vi "ConvolveFile.vi"(11 "Old Files":T1[](array[typedef])) -> ()   [LabVIEW 2025]
uses:
  Curtin1_Label.ctl
panel:
  in  "Save":bool=TRUE
  out "ratio":dbl format="%0.2e"
  in  "Musical Piece":enum32{"Default", "Advanced"}(tab)
  in  "Path":path
  in  "Play 3":bool
  in  "Sampling rate":u16=48000
  out "FRF":cluster{"t0":dbl, "dt":dbl, dbl[]}[](graph)=[{"t0"=0.0, "dt"=0.732421875, array[13995 elements]}, {"t0"=0.0, "dt"=0.732421875, array[13995 elements]}]
  out "PointIdx":i32=359
  out "CursLoc":cluster{"X":dbl, "Y":dbl}={"X"=262.939453125, "Y"=26.045098132964196}
  out "CursIdx":i32=1
  in  "Play 2":bool
  in  "Play":bool
  in  "Save Convolve":bool
  in  "Instruments":u16(ring) items=["1727 Kreutzer Vengerov Strad 01 H.AvC"]
  # "Left ear is original\nRight ear is modified"
  # "Tchaikovsky Violin Concerto run"
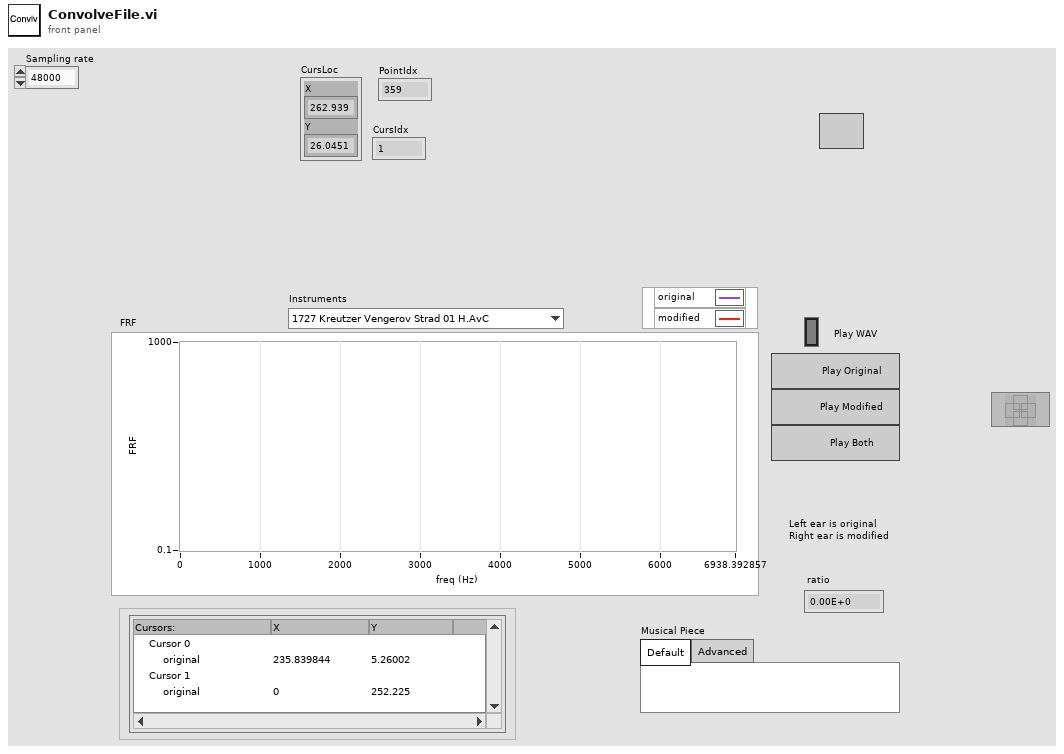
[diagram p1: front panel]
types:
  T1 = typedef "Curtin1_Label.ctl" = cluster{"Show?":bool, "Name":string, "Color":u32, "Path":path, "Show Notes":bool}
  T2 = typedef "PreferencesControl.ctl" = cluster{"Name of test":string, "Date":timestamp, "Location":string, "Template":string, "Soundcard":string, "resolution":u16, "Sampling rate":u16, "Ch1 Gain ":dbl, "Ch2 Gain":dbl, "Sample time (s)":dbl, "Pre-trigger (s)":dbl, "Hammer Threshold":dbl, "Positions":i16, "Taps/Position":i16, "Set Names":string, "Freq resolution":dbl, "Hammer cutoff":dbl, "Mic cutoff":dbl, "Double bounce ":dbl, "Hammer Cal":dbl, "dB Offset":dbl, "Accel Cal":dbl, "Vibrometer Cal":dbl, "Mic Cal":dbl, "Output":u16, "Voltage Cal":dbl, "Vibrometer Port":refnum<visa-resource-name>, "Range":u16, "High Pass":u16, "Bandwidth":u16, "X Range":cluster{"Minimum":dbl, "Maximum":dbl, "Increment":dbl, "Minor Increment":dbl, "Start":dbl}[], "Y Range":cluster{"Minimum":dbl, "Maximum":dbl, "Increment":dbl, "Minor Increment":dbl, "Start":dbl}[], "dB Spread":dbl, "Trigger":u16, "Ch_1":u8, "Ch_2":u8, "flip?":bool, "60Hz":bool, "Time offset":dbl, "Piezo Cal":dbl, "Default Notes":string, "Tom":bool}
  T3 = typedef "LVCursorListTypeDef.ctl" = cluster{"Name":string, "Color":u32, "Style":u8, "Point Style":u8, "Name Visible":bool, "Allow Drag":bool, "Cursor Mode":u32, "Plot":i32, "Index":i32, "Position":cluster{"X":dbl, "Y":dbl}, "X Scale":u32, "Y Scale":u32, "Watch Plots":i32[], "Watch All Plots":bool, "Plot Area":i32, "Label Offset":cluster{"X":dbl, "Y":dbl}}[]
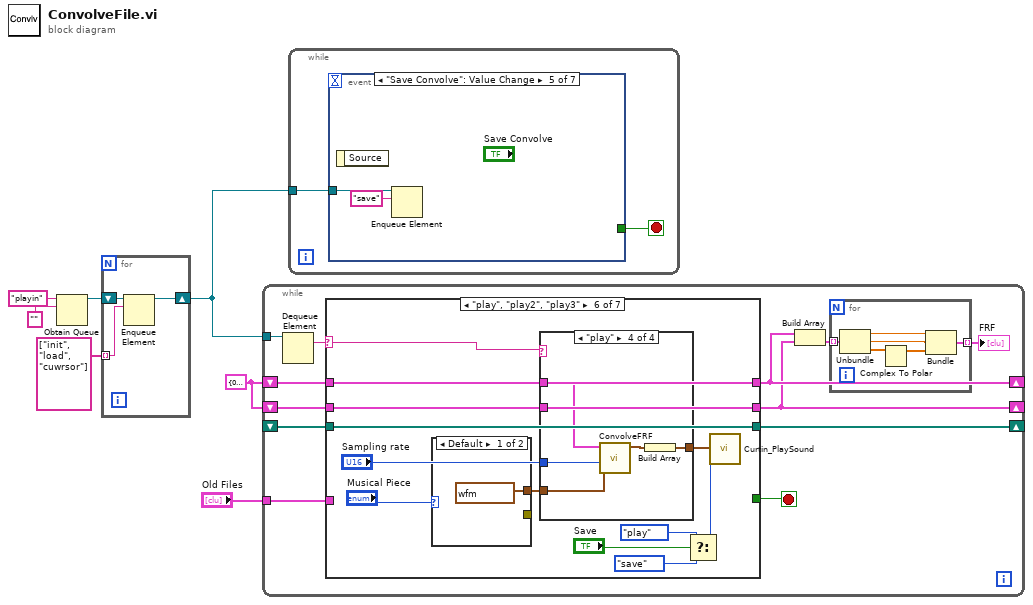
[diagram p0: block diagram]
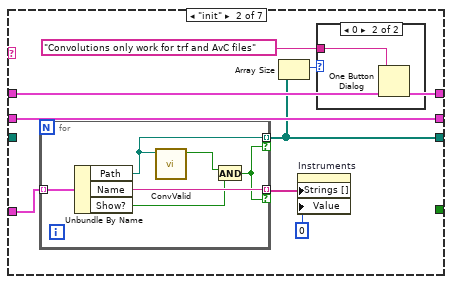
[diagram p3: hidden frame]
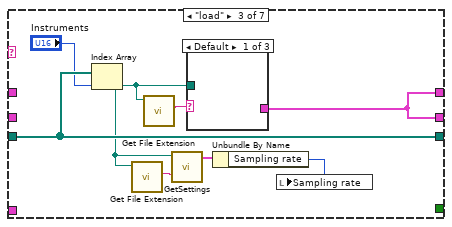
[diagram p5: hidden frame]
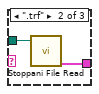
[diagram p6: hidden frame]
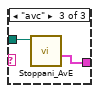
[diagram p7: hidden frame]
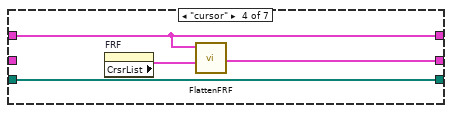
[diagram p8: hidden frame]
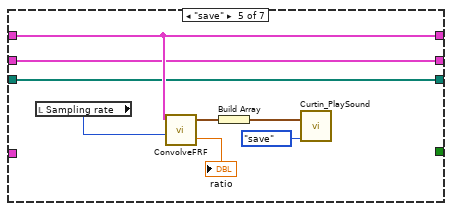
[diagram p9: hidden frame]
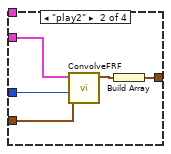
[diagram p11: hidden frame]
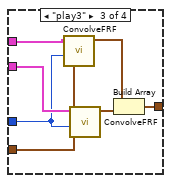
[diagram p12: hidden frame]
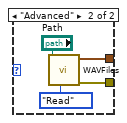
[diagram p13: hidden frame]
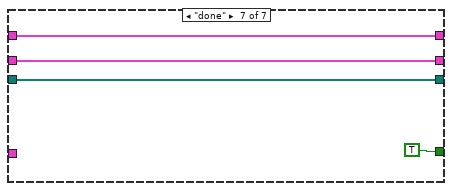
[diagram p14: hidden frame]
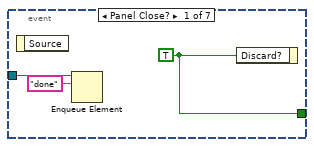
[diagram p15: hidden frame]
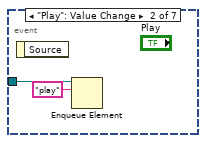
[diagram p16: hidden frame]
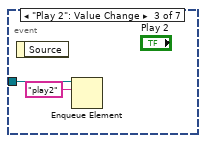
[diagram p17: hidden frame]
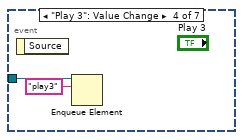
[diagram p18: hidden frame]
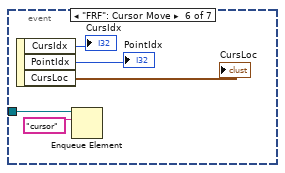
[diagram p19: hidden frame]
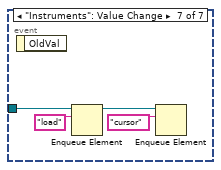
[diagram p20: hidden frame]
diagram:
  w1 = cluster{"t0":dbl, "dt":dbl, "Y":cdb[]} {"t0"=0.0, "dt"=0.0, "Y"=[]} ("Complex FRF")
  n1 = Obtain Queue(name (unnamed)="playin", element data type="" ("element")) -> (queue out=w7:refnum<queue>)  [unwired: 3 in, 2 out]
  n2 = for {
    shift-right: [w9] -> w6
    shift-left: w7 -> [w10]
    tunnel: string[] ["init", "load", "cuwrsor"] -> [w8] mode=indexing
    n3 = Enqueue Element(queue=w10, element=w8) -> (queue out=w9:refnum<queue>)  [unwired: 2 in, 2 out]
  }
  n4 = while {
    tunnel: w6 -> [w22]
    shift-right: [w16] -> _
    shift-left: w1 -> [w19]
    shift-right: [w15] -> _
    shift-left: w1 -> [w18]
    tunnel: "Old Files" -> [w13]
    shift-right: [w12] -> _
    shift-left: _ -> [w11]
    stop <- w20 stop-if-true
    n5 = Dequeue Element(queue=w22) -> (element=w21:string)  [unwired: 2 in, 3 out]
    n6 = case shown="\"play\", \"play2\", \"play3\"" w21 {
      selector: w21 -> [_ _ _ _ _ w76 _]
      tunnel: [_ _ _ _ _ _ TRUE] -> w20
      tunnel: [w31 w39 w54 w61 w69 w75 w107] -> w16
      tunnel: w19 -> [w31 w39 _ w61 w69 w75 w107]
      tunnel: w18 -> [w30 w38 _ _ w67 w80 w106]
      tunnel: [w30 w38 w54 w59 w67 w80 w106] -> w15
      tunnel: w13 -> [_ w35 _ _ _ _ _]
      tunnel: [w29 w34 w53 w62 w66 w79 w105] -> w12
      tunnel: w11 -> [w29 _ w53 w62 w66 w79 w105]
      frame Default {
      }
      frame "init" {
        n7 = for {
          tunnel: [w46] -> w37 mode=indexing if=w42
          tunnel: [w44] -> w34 mode=indexing if=w42
          tunnel: w35 -> [w45] mode=indexing
          n8 = Unbundle By Name(w45) -> ("Path"=w44:path, "Name"=w46:string, "Show?"=w43:bool)
          n9 = call "ConvValid.vi"("Path"=w44) -> ("Valid"=w41:bool)  [unwired: 10 in]
          n10 = And(x=w41, y=w43) -> (x .and. y?=w42:bool)
        }
        n11 = Array Size(array=w34) -> (size(s)=w33:i32)
        n12 = property on="Instruments" class="Ring (strict)"("Strings []"=w37, "Value"=0) -> ()  [unwired: 2 in, 2 out]
        n13 = case shown="0" w33 {
          tunnel: "Convolutions only work for trf and AvC files" ("element") -> [_ w40]
          frame Default {
          }
          frame 0 {
            n14 = One Button Dialog(message=w40) -> ()  [unwired: 1 in, 1 out]
          }
        }
      }
      frame "load" {
        n15 = Index Array(array=w53, index="Instruments") -> (element=w48:path)
        n16 = call <vilib>:"Get File Extension.vi"("file"=w48) -> ("lowercase file extension"=w52:string)  [unwired: 6 in, 4 out]
        n17 = call <vilib>:"Get File Extension.vi"("file"=w48) -> ("lowercase file extension"=w47:string)  [unwired: 6 in, 4 out]
        n18 = call "GetSettings.vi"("lowercase file extension"=w52, "wavform file"=w48) -> ("Settings"=w51:T2)  [unwired: 8 in, 1 out]
        n19 = case shown="Default" w47 {
          tunnel: [_ w56 w57] -> w54
          tunnel: w48 -> [_ w55 w58]
          frame Default {
          }
          frame ".trf" {
            n20 = call "Stoppani File Read.vi"("String in"=w55) -> ("Complex FRF"=w56:cluster{"t0":dbl, "dt":dbl, "Y":cdb[]})  [unwired: 2 in, 3 out]
          }
          frame "avc" {
            n21 = call "Stoppani_AvE.vi"("file (use dialog)"=w58) -> ("Complex FRF"=w57:cluster{"t0":dbl, "df":dbl, "Y":cdb[]})  [unwired: 7 in, 3 out]
          }
        }
        n22 = Unbundle By Name(w51) -> ("Sampling rate"=w50:u16)
        n23 = local write "Sampling rate"(w50) -> ()
      }
      frame "cursor" {
        n24 = property on="FRF" class="WFGraph (strict)"() -> ("CrsrList"=w60:T3)  [unwired: 2 in, 2 out]
        n25 = call "FlattenFRF.vi"("CrsrList"=w60, "Complex FRF in"=w61) -> ("Complex FRF out"=w59:cluster{"t0":dbl, "dt":dbl, "Y":cdb[]})  [unwired: 9 in]
      }
      frame "save" {
        n26 = local read "Sampling rate"() -> (w65:u16)
        n27 = call "ConvolveFRF.vi"("Sampling rate"=w65, "Complex FRF"=w69) -> ("Convolution"=w68:waveform(dbl), "ratio"=→"ratio":dbl)  [unwired: 6 in, 2 out]
        n28 = Build Array(w68) -> (w70:waveform(dbl)[])
        n29 = call "Curtin_PlaySound.vi"("Task"=enum16{"play", "save"}."save", "all waveforms"=w70) -> ()  [unwired: 9 in, 1 out]
      }
      frame "play", "play2", "play3" {
        n30 = case shown="Default" "Musical Piece" {
          tunnel: [waveform(dbl)[] [{"t0"=timestamp(0 s since 1904-01-01), "dt"=2.0833333333333333e-05, "Y"=array[288010 elements]}, {"t0"=timestamp(0 s since 1904-01-01), "dt"=2.0833333333333333e-05, "Y"=array[288010 elements]}] ("musical piece") w103] -> w78
          tunnel: [_ w101] -> _
          frame Default {
          }
          frame "Advanced" {
            n31 = call "WAVFiles.vi"("Task"=enum16{"Read", "Write", "wfm"}."Read", "WAV File"="Path") -> ("error out"=w101:errorcluster, "Data"=w103:waveform(dbl)[])  [unwired: 6 in, 2 out]
          }
        }
        n32 = case shown="\"play\"" w76 {
          tunnel: [_ w87 w94 w99] -> w82
          tunnel: "Sampling rate" -> [_ w86 w90 w98]
          tunnel: w80 -> [_ w85 w93 _]
          tunnel: w78 -> [_ w83 w89 w96]
          tunnel: w75 -> [_ _ w91 w95]
          frame Default {
          }
          frame "play2" {
            n33 = call "ConvolveFRF.vi"("musical piece"=w83, "Sampling rate"=w86, "Complex FRF"=w85) -> ("Convolution"=w84:waveform(dbl))  [unwired: 5 in, 3 out]
            n34 = Build Array(w84) -> (w87:waveform(dbl)[])
          }
          frame "play3" {
            n35 = call "ConvolveFRF.vi"("musical piece"=w89, "Sampling rate"=w90, "Complex FRF"=w91) -> ("Convolution"=w88:waveform(dbl))  [unwired: 5 in, 3 out]
            n36 = call "ConvolveFRF.vi"("musical piece"=w89, "Sampling rate"=w90, "Complex FRF"=w93) -> ("Convolution"=w92:waveform(dbl))  [unwired: 5 in, 3 out]
            n37 = Build Array(w88, w92) -> (w94:waveform(dbl)[])
          }
          frame "play" {
            n38 = call "ConvolveFRF.vi"("musical piece"=w96, "Sampling rate"=w98, "Complex FRF"=w95) -> ("Convolution"=w97:waveform(dbl))  [unwired: 5 in, 3 out]
            n39 = Build Array(w97) -> (w99:waveform(dbl)[])
          }
        }
        n40 = Select(t=enum16{"play", "save"}."play" ("Task"), s="Save", f=enum16{"play", "save"}."save" ("Task")) -> (s? t:f=w71:enum16{"play", "save"})
        n41 = call "Curtin_PlaySound.vi"("Task"=w71, "all waveforms"=w82) -> ()  [unwired: 9 in, 1 out]
      }
      frame "done" {
      }
    }
    n42 = Build Array(w16, w15) -> (w14:cluster{"t0":dbl, "dt":dbl, "Y":cdb[]}[])
    n43 = for {
      tunnel: [w26] -> w17 mode=indexing
      tunnel: w14 -> [w23] mode=indexing
      n44 = Unbundle(w23) -> ("t0"=w28:dbl, "dt"=w27:dbl, "Y"=w24:cdb[])
      n45 = Complex To Polar(r * e^(i*theta)=w24) -> (r=w25:dbl[])  [unwired: 1 out]
      n46 = Bundle("t0"=w28, "dt"=w27, w25) -> (w26:cluster{"t0":dbl, "dt":dbl, dbl[]})  [unwired: 1 in]
    }
    "FRF" <- w17
  }
  n47 = while {
    tunnel: w6 -> [w110]
    stop <- w109 stop-if-true
    n48 = event shown="[4] \"Save Convolve\": Value Change" {
      selector: _ -> [_ _ _ _ _ _ _]
      dyn-events: _ -> [_ _ _ _ _ _ _]
      timeout: _ -> [_ _ _ _ _ _ _]
      tunnel: w110 -> [w113 w115 w117 w119 w121 w126 w130]
      tunnel: [w112 _ _ _ _ _ _] -> w109
      event Panel Close? {
        w112 = TRUE ("Discard?")
        n49 = event-data() -> ()  [unwired: 1 in, 1 out]
        n50 = Enqueue Element(queue=w113, element="done") -> ()  [unwired: 2 in, 3 out]
        n51 = event-data("Discard?"=w112) -> ()  [unwired: 1 in, 1 out]
      }
      event "Play": Value Change {
        n52 = event-data() -> ()  [unwired: 1 in, 1 out]
        n53 = Enqueue Element(queue=w115, element="play") -> ()  [unwired: 2 in, 3 out]
      }
      event "Play 2": Value Change {
        n54 = event-data() -> ()  [unwired: 1 in, 1 out]
        n55 = Enqueue Element(queue=w117, element="play2") -> ()  [unwired: 2 in, 3 out]
      }
      event "Play 3": Value Change {
        n56 = event-data() -> ()  [unwired: 1 in, 1 out]
        n57 = Enqueue Element(queue=w119, element="play3") -> ()  [unwired: 2 in, 3 out]
      }
      event "Save Convolve": Value Change {
        n58 = event-data() -> ()  [unwired: 1 in, 1 out]
        n59 = Enqueue Element(queue=w121, element="save") -> ()  [unwired: 2 in, 3 out]
      }
      event "FRF": Cursor Move {
        n60 = event-data() -> ("CursIdx"=→"CursIdx":i32, "PointIdx"=→"PointIdx":i32, "CursLoc"=→"CursLoc":cluster{"X":dbl, "Y":dbl})  [unwired: 1 in]
        n61 = Enqueue Element(queue=w126, element="cursor") -> ()  [unwired: 2 in, 3 out]
      }
      event "Instruments": Value Change {
        n62 = event-data() -> ()  [unwired: 1 in, 1 out]
        n63 = Enqueue Element(queue=w130, element="load") -> (queue out=w127:refnum<queue>)  [unwired: 2 in, 2 out]
        n64 = Enqueue Element(queue=w127, element="cursor") -> ()  [unwired: 2 in, 3 out]
      }
    }
  }
